vi "Trial v0.vi"(2 "error in (no error)":errorcluster, 3 "queue in":refnum<queue>, 4 "DDA":bool=TRUE) -> (0 "error out":errorcluster={"status"=TRUE, "code"=1, "source"="Enqueue Element in Trial.vi"}, 1 "queue out":refnum<queue>)   [LabVIEW 2017]
uses:
  SubVI/Global.vi
  <vilib>/Analysis/NI_AALPro.lvlib
  <vilib>/robotics/Kinematics/NI_Kinematics.lvlib
  Control/RPY.ctl
  Control/State.ctl
  <vilib>/Analysis/NI_AALBase.lvlib
  <vilib>/Analysis/baseanly.llb/Real Dot Product.vi
  <vilib>/Analysis/_algsub.llb/Real Vector Norm.vi
panel:
  in  "alpha theta":dbl=1.0
  in  "lambda theta":dbl=1.0
  in  "alpha w":dbl=1.0
  in  "lambda w":dbl=1.0
  in  "alpha Rbar":dbl=1.0
  in  "n":i32=2
  in  "Time Target (s)":dbl=10.0
  in  "epsilon":dbl=0.1
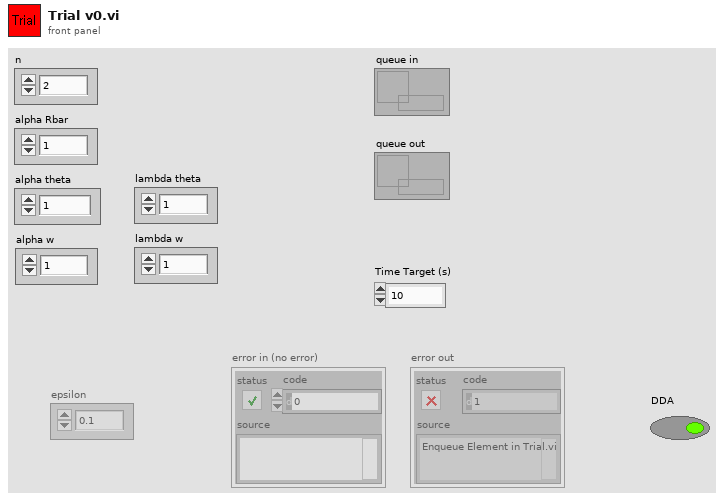
[diagram p1: front panel]
types:
  T1 = typedef "State.ctl" = cluster{"Inertia (Kg)":dbl, "Damping (N*s/m)":dbl, "RoM (deg)":dbl}
  T2 = typedef "RPY.ctl" = cluster{"roll":dbl, "pitch":dbl, "yaw":dbl}
  T3 = typedef "NI_Matrix.lvlib/RealMatrix.ctl" = dbl[][]
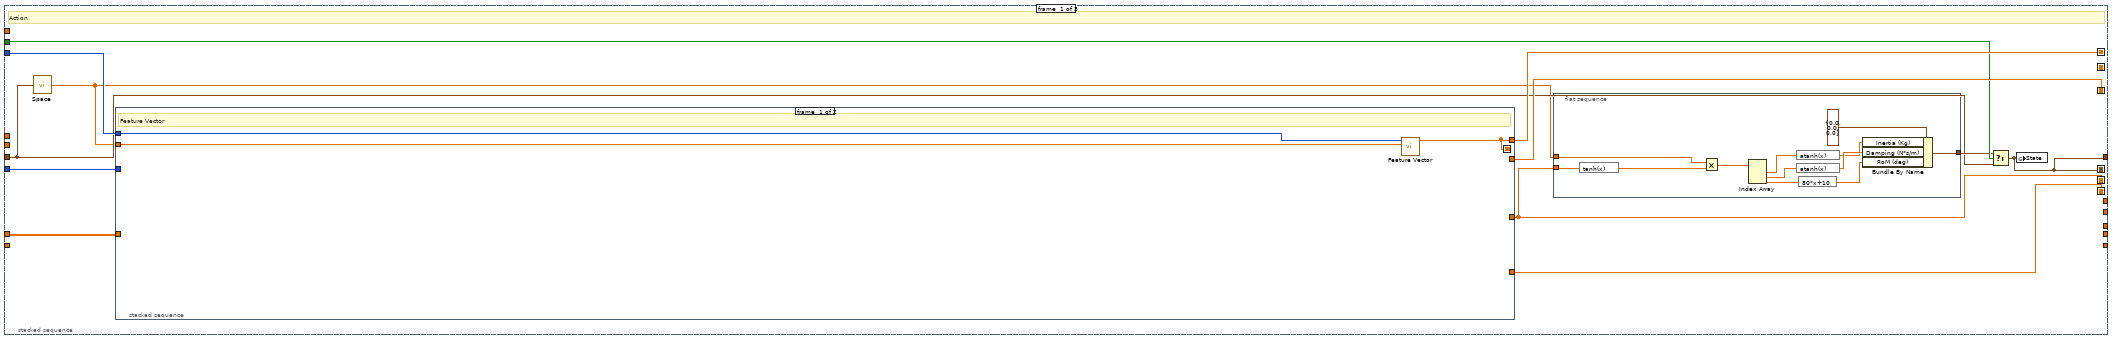
[diagram p7: hidden frame]
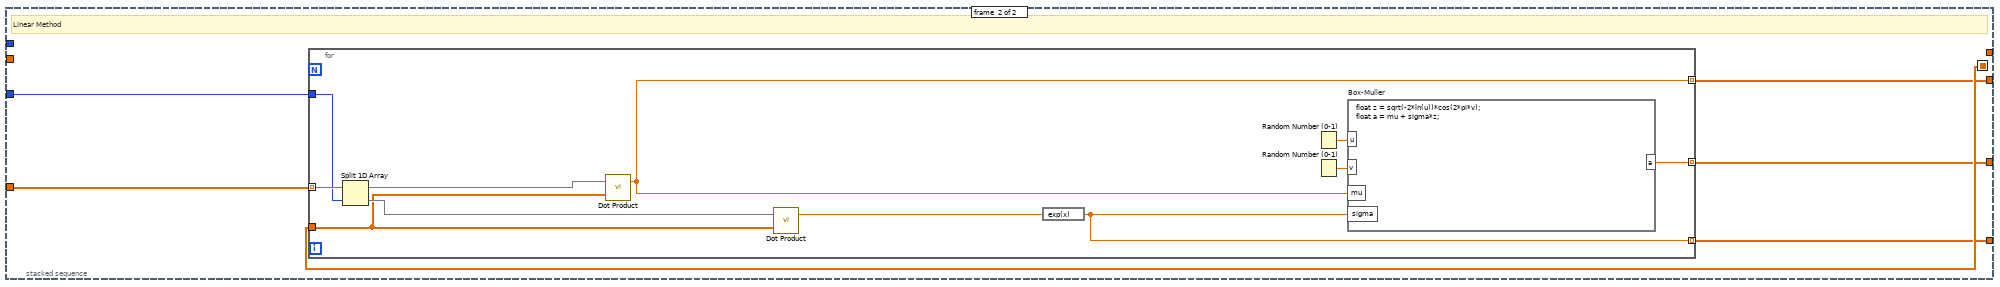
[diagram p8: hidden frame]
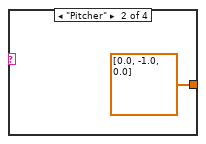
[diagram p9: hidden frame]
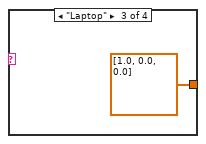
[diagram p10: hidden frame]
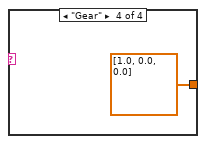
[diagram p11: hidden frame]
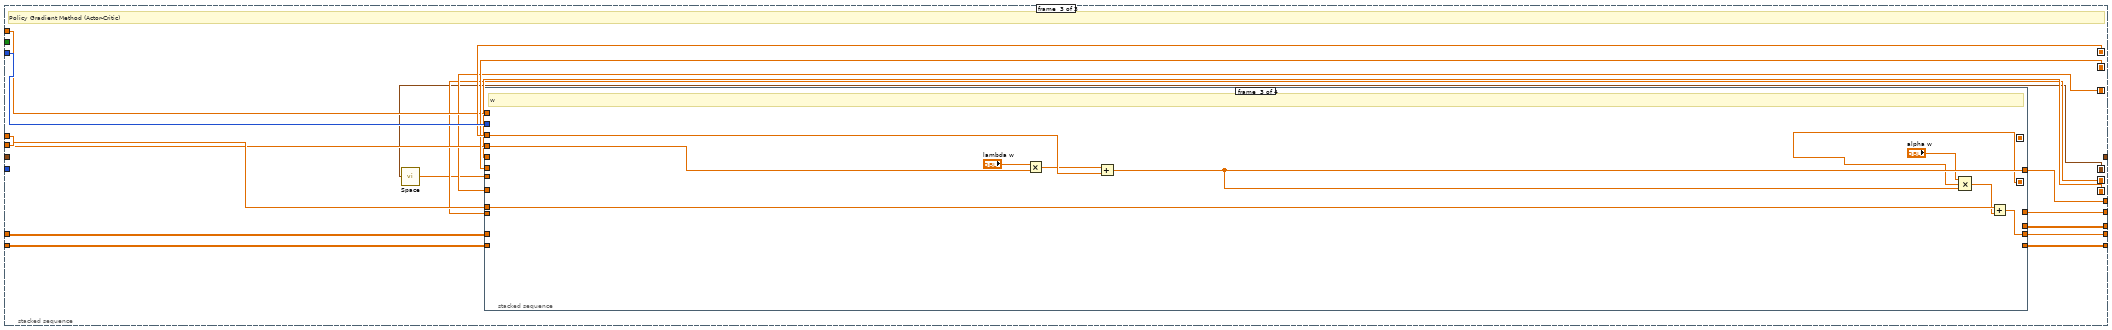
[diagram p12: hidden frame]
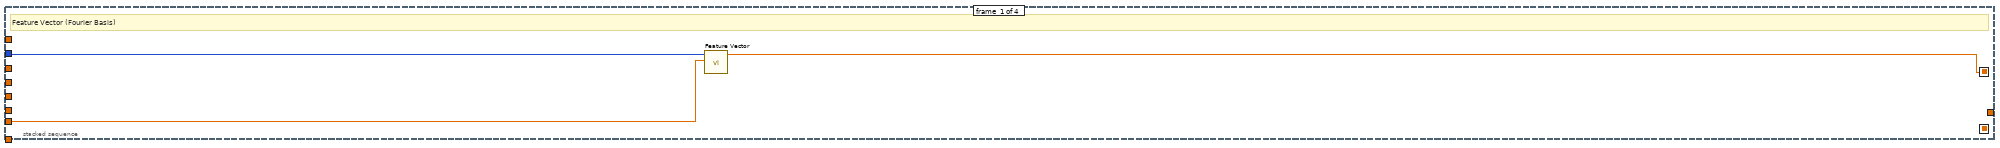
[diagram p13: hidden frame]
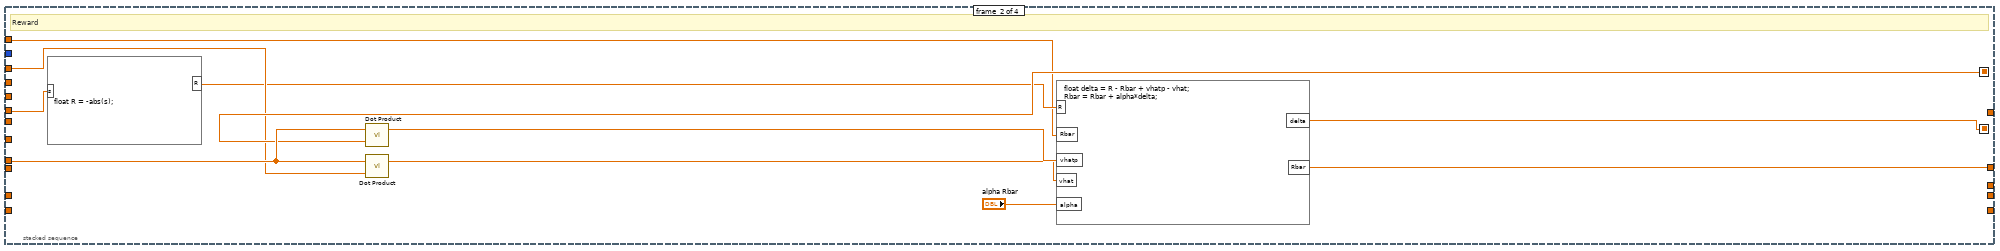
[diagram p14: hidden frame]
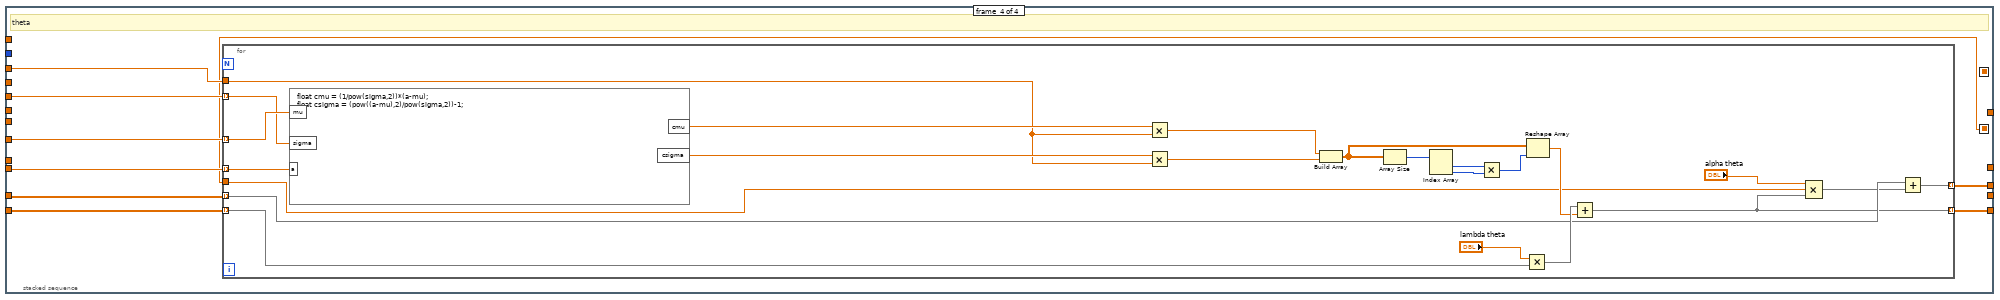
[diagram p15: hidden frame]
diagram:
  n1 = flat-sequence {
    tunnel: [w9] -> w5
    tunnel: "error in (no error)" -> [w10]
    tunnel: "queue in" -> [w8]
    tunnel: "DDA" -> [w11]
    tunnel: [w7] -> w1
    frame #0 {
      w14 = 0.0  # Rbar
      n2 = Increment(x="n") -> (x+1=w18:i32)
      n3 = expression code="2*pow(x,3)"(w18) -> (w20:i32)
      n4 = Initialize Array(0.0 ("element"), 3 ("dimension size"), w20) -> (w12:dbl[][])
      n5 = expression code="pow(x,3)"(w18) -> (w15:i32)
      n6 = Initialize Array(0.0 ("element"), w15) -> (w13:dbl[])
      n7 = global read "Global.vi" "State"() -> (w6:T1)
      n8 = while {
        shift-right: [w37] -> _
        shift-left: w6 -> [w41]
        shift-right: [w28] -> _
        shift-left: w12 -> [w39]
        tunnel: w18 -> [w40]
        tunnel: w15 -> [w38]
        shift-right: [w31] -> _
        shift-left: w13 -> [w36]
        shift-right: [w34] -> _
        shift-left: w14 -> [w35]
        shift-right: [w32] -> _
        shift-left: w13 -> [w33]
        shift-right: [w29] -> _
        shift-left: w12 -> [w30]
        tunnel: w11 -> [w27]
        shift-right: [w23] -> w7
        shift-left: w8 -> [w25]
        shift-right: [w22] -> w9
        shift-left: w10 -> [w26]
        stop <- w42 stop-if-true
        # "Multiple Trials"
        n9 = stacked-sequence {
          seq-local: [w50 _ _] -> [_ w89 w144]
          seq-local: [_ w90 _] -> [_ _ w157]
          seq-local: [w51 _ _] -> [_ _ w159]
          seq-local: [w49 _ _] -> [_ _ w150]
          seq-local: [w48 _ _] -> [_ _ w149]
          seq-local: [w43 _ _] -> [_ _ w148]
          tunnel: w41 -> [w45 _ _]
          tunnel: w40 -> [w54 _ w160]
          tunnel: w39 -> [w53 _ w146]
          tunnel: w38 -> [w52 _ _]
          tunnel: [w50 _ _] -> w37
          tunnel: w36 -> [_ _ w158]
          tunnel: w35 -> [_ _ w156]
          tunnel: [_ _ w155] -> w34
          tunnel: w33 -> [_ _ w154]
          tunnel: [_ _ w153] -> w32
          tunnel: [_ _ w152] -> w31
          tunnel: w30 -> [_ _ w151]
          tunnel: [_ _ w147] -> w29
          tunnel: [_ _ w145] -> w28
          tunnel: w27 -> [w47 _ _]
          frame #0 {
            # "Action"
            n10 = call "Space.vi"("State"=w45) -> ("Array"=w44:dbl[])
            n11 = stacked-sequence {
              seq-local: [w67 _] -> [_ w73]
              tunnel: w54 -> [w69 _]
              tunnel: w53 -> [_ w75]
              tunnel: w52 -> [_ w74]
              tunnel: w44 -> [w68 _]
              tunnel: [w67 _] -> w51
              tunnel: [_ w72] -> w49
              tunnel: [_ w71] -> w48
              tunnel: [_ w70] -> w43
              frame #0 {
                # "Feature Vector"
                n12 = call "Feature Vector.vi"("state"=w68, "n"=w69) -> ("vector"=w67:dbl[])  [unwired: 9 in]
              }
              frame #1 {
                # "Linear Method"
                n13 = for {
                  tunnel: w75 -> [w84] mode=indexing
                  tunnel: w74 -> [w83]
                  tunnel: w73 -> [w80]
                  tunnel: [w78] -> w70 mode=indexing
                  tunnel: [w77] -> w72 mode=indexing
                  tunnel: [w76] -> w71 mode=indexing
                  n14 = Split 1D Array(array=w84, index=w83) -> (first subarray=w82:dbl[], second subarray=w81:dbl[])
                  n15 = call-poly <vilib>:"Dot Product.vi"("Y Vector"=w80, "X Vector"=w82) -> ("X * Y"=w77:dbl)  [unwired: 1 out]
                  n16 = call-poly <vilib>:"Dot Product.vi"("Y Vector"=w80, "X Vector"=w81) -> ("X * Y"=w79:dbl)  [unwired: 1 out]
                  n17 = expression code="exp(x)"(w79) -> (w76:dbl)
                  n18 = Random Number (0-1)() -> (number: 0 to 1=w86:dbl)
                  n19 = Random Number (0-1)() -> (number: 0 to 1=w85:dbl)
                  n20 = formula code="float z = sqrt(-2*ln(u))*cos(2*pi*v);\nfloat a = mu + sigma*z;" "Box-Muller"("u"=w86, "v"=w85, "mu"=w77, "sigma"=w76) -> ("a"=w78:dbl)
                }
              }
            }
            n21 = flat-sequence {
              tunnel: [w66] -> w46
              tunnel: w44 -> [w65]
              tunnel: w43 -> [w56]
              frame #0 {
                n22 = expression code="tanh(x)"(w56) -> (w64:dbl[])
                n23 = Multiply(x=w65, y=w64) -> (x*y=w63:dbl[])
                n24 = Index Array(array=w63) -> (element #1=w58:dbl, element #2=w60:dbl, element #3=w62:dbl)  [unwired: 3 in]
                n25 = expression code="atanh(x)"(w58) -> (w57:dbl)
                n26 = expression code="atanh(x)"(w60) -> (w59:dbl)
                n27 = expression code="80*x+10"(w62) -> (w61:dbl)
                n28 = Bundle By Name(cluster=T1 {"Inertia (Kg)"=0.0, "Damping (N*s/m)"=0.0, "RoM (deg)"=0.0} ("State"), "Inertia (Kg)"=w57, "Damping (N*s/m)"=w59, "RoM (deg)"=w61) -> (w66:T1)
              }
            }
            n29 = Select(t=w46, s=w47, f=w45) -> (s? t:f=w50:T1)
            n30 = global write "Global.vi" "State"(w50) -> ()
          }
          frame #1 {
            # "Observation"
            n31 = global read "Global.vi" "ADL"() -> (w92:string)
            n32 = case shown="\"Book\", Default" w92 {
              tunnel: [dbl[] [0.0, 1.0, 0.0] dbl[] [0.0, -1.0, 0.0] dbl[] [1.0, 0.0, 0.0] dbl[] [1.0, 0.0, 0.0]] -> w91
              frame "Book", Default {
              }
              frame "Pitcher" {
              }
              frame "Laptop" {
              }
              frame "Gear" {
              }
            }
            n33 = Unbundle By Name(w89) -> ("RoM (deg)"=w88:dbl)
            n34 = expression code="(x/180.0)*pi" "degrees to radians"(w88) -> (w87:dbl)
            n35 = call <vilib>:"Angle Vector to Rotation Matrix.vi"("vector"=w91, "angle"=w87) -> ("rotation matrix"=w95:T3)
            n36 = call <vilib>:"Rotation Matrix to Roll Pitch Yaw.vi"("rotation matrix"=w95) -> ("angles"=w96:cluster{"roll":dbl, "pitch":dbl, "yaw":dbl})
            n37 = Unbundle By Name(w96) -> ("roll"=w97:dbl, "pitch"=w98:dbl, "yaw"=w99:dbl)
            n38 = Bundle By Name(cluster=T2 {"roll"=0.0, "pitch"=0.0, "yaw"=0.0} ("Target"), "roll"=w97, "pitch"=w98, "yaw"=w99) -> (w93:T2)
            n39 = while {
              tunnel: w93 -> [w115]
              shift-right: [w107] -> _
              shift-left: 0.0 -> [w108]
              tunnel: [w106] -> _
              tunnel: [w105] -> w90
              i -> [w118]
              stop <- w111 stop-if-true
              # "1 Trial"
              n40 = Quotient & Remainder(x=w118, y=2) -> (x-y*floor(x/y)=w116:i32)  [unwired: 1 out]
              n41 = Equal To 0?(x=w116) -> (x = 0?=w110:bool)
              n42 = Not(x=w110) -> (.not. x?=w109:bool)
              n43 = global read "Global.vi" "Stop"() -> (w112:bool)
              n44 = Select(t=w115, s=w110, f=T2 {"roll"=0.0, "pitch"=0.0, "yaw"=0.0} ("Target")) -> (s? t:f=w113:T2)
              n45 = global write "Global.vi" "Target"(w113) -> ()
              n46 = Or(x=w109, y=w112) -> (x .or. y?=w111:bool)
              n47 = call <vilib>:"High Resolution Relative Seconds.vi"() -> ("relative seconds"=w120:dbl)
              n48 = while {
                tunnel: w113 -> [w127]
                shift-right: [w133] -> _
                shift-left: w120 -> [w134]
                shift-right: [w125] -> _
                shift-left: 0.0 -> [w132]
                tunnel: w108 -> [w126]
                tunnel: [w123] -> w107
                tunnel: ["epsilon"] -> w106
                tunnel: [w122] -> w105
                stop <- w135 stop-if-true
                # "1/2 Trial"
                n49 = Wait (ms)(milliseconds to wait=u32 10) -> ()  [unwired: 1 out]
                n50 = global read "Global.vi" "Object"() -> (w140:T2)
                n51 = call <vilib>:"High Resolution Relative Seconds.vi"() -> ("relative seconds"=w133:dbl)
                n52 = global read "Global.vi" "Playback"() -> (w131:bool)
                n53 = Subtract(x=w140, y=w127) -> (x-y=w141:T2)
                n54 = Subtract(x=w133, y=w134) -> (x-y=w130:dbl)
                n55 = Cluster To Array(cluster=w141) -> (array=w142:dbl[])
                n56 = Select(t=w130, s=w131, f=0.0) -> (s? t:f=w129:dbl)
                n57 = call-poly <vilib>:"Vector Norm.vi"("Input Vector"=w142) -> ("norm"=w139:dbl)  [unwired: 9 in, 1 out]
                n58 = Add(x=w129, y=w132) -> (x+y=w125:dbl)
                n59 = Less?(x=w139, y="epsilon") -> (x < y?=w138:bool)
                n60 = Add(x=w125, y=w126) -> (x+y=w123:dbl)
                n61 = global read "Global.vi" "Stop"() -> (w137:bool)
                n62 = Subtract(x="Time Target (s)", y=w123) -> (x-y=w122:dbl)
                n63 = global write "Global.vi" "Score"(w122) -> ()
                n64 = Or(x=w138, y=w137) -> (x .or. y?=w135:bool)
              }
            }
          }
          frame #2 {
            # "Policy Gradient Method (Actor-Critic)"
            n65 = call "Space.vi"("State"=w144) -> ("Array"=w143:dbl[])
            n66 = stacked-sequence {
              seq-local: [w161 _ _ _] -> [_ w173 _ _]
              seq-local: [_ w164 _ _] -> [_ _ w177 w185]
              tunnel: w143 -> [w163 _ _ _]
              tunnel: w160 -> [w162 _ _ _]
              tunnel: w159 -> [_ w172 w184 w189]
              tunnel: w158 -> [_ w174 w180 _]
              tunnel: w157 -> [_ w169 _ _]
              tunnel: w156 -> [_ w167 _ _]
              tunnel: [_ w165 _ _] -> w155
              tunnel: w154 -> [_ _ w183 _]
              tunnel: [_ _ w178 _] -> w153
              tunnel: [_ _ w175 _] -> w152
              tunnel: w151 -> [_ _ _ w193]
              tunnel: w150 -> [_ _ _ w192]
              tunnel: w149 -> [_ _ _ w191]
              tunnel: w148 -> [_ _ _ w190]
              tunnel: [_ _ _ w188] -> w147
              tunnel: w146 -> [_ _ _ w187]
              tunnel: [_ _ _ w186] -> w145
              frame #0 {
                # "Feature Vector (Fourier Basis)"
                n67 = call "Feature Vector.vi"("state"=w163, "n"=w162) -> ("vector"=w161:dbl[])  [unwired: 9 in]
              }
              frame #1 {
                # "Reward"
                n68 = formula code="float R = -abs(s);"("s"=w169) -> ("R"=w168:dbl)
                n69 = call-poly <vilib>:"Dot Product.vi"("Y Vector"=w173, "X Vector"=w174) -> ("X * Y"=w171:dbl)  [unwired: 1 out]
                n70 = call-poly <vilib>:"Dot Product.vi"("Y Vector"=w172, "X Vector"=w174) -> ("X * Y"=w170:dbl)  [unwired: 1 out]
                n71 = formula code="float delta = R - Rbar + vhatp - vhat;\nRbar = Rbar + alpha*delta;"("R"=w168, "Rbar"=w167, "vhatp"=w171, "vhat"=w170, "alpha"="alpha Rbar") -> ("delta"=w164:dbl, "Rbar"=w165:dbl)
              }
              frame #2 {
                # "w"
                n72 = Multiply(x="lambda w", y=w183) -> (x*y=w181:dbl[])
                n73 = Add(x=w181, y=w184) -> (x+y=w178:dbl[])
                n74 = Compound Arithmetic op=MULTIPLY("alpha w", w177, w178) -> (w179:dbl[])
                n75 = Add(x=w180, y=w179) -> (x+y=w175:dbl[])
              }
              frame #3 {
                # "theta"
                n76 = for {
                  tunnel: w193 -> [w215] mode=indexing
                  tunnel: w192 -> [w213] mode=indexing
                  tunnel: w191 -> [w212] mode=indexing
                  tunnel: w190 -> [w211] mode=indexing
                  tunnel: w189 -> [w208]
                  tunnel: [w198] -> w188 mode=indexing
                  tunnel: w187 -> [w203] mode=indexing
                  tunnel: [w201] -> w186 mode=indexing
                  tunnel: w185 -> [w199]
                  n77 = formula code="float cmu = (1/pow(sigma,2))*(a-mu);\nfloat csigma = (pow((a-mu),2)/pow(sigma,2))-1;"("mu"=w213, "sigma"=w212, "a"=w211) -> ("cmu"=w210:dbl, "csigma"=w209:dbl)
                  n78 = Multiply(x=w210, y=w208) -> (x*y=w207:dbl[])
                  n79 = Multiply(x=w209, y=w208) -> (x*y=w206:dbl[])
                  n80 = Build Array(w207, w206) -> (w197:dbl[][])
                  n81 = Array Size(array=w197) -> (size(s)=w205:i32[])
                  n82 = Index Array(array=w205) -> (element #1=w196:i32, element #2=w195:i32)  [unwired: 2 in]
                  n83 = Multiply(x=w196, y=w195) -> (x*y=w194:i32)
                  n84 = Multiply(x="lambda theta", y=w215) -> (x*y=w214:dbl[])
                  n85 = Reshape Array(w197, w194) -> (w204:dbl[])
                  n86 = Add(x=w214, y=w204) -> (x+y=w198:dbl[])
                  n87 = Compound Arithmetic op=MULTIPLY("alpha theta", w199, w198) -> (w202:dbl[])
                  n88 = Add(x=w203, y=w202) -> (x+y=w201:dbl[])
                }
              }
            }
          }
        }
        n89 = Enqueue Element(queue=w25, element="", error in (no error)=w26) -> (queue out=w23:refnum<queue>, error out=w22:errorcluster)  [unwired: 1 in, 1 out]
        n90 = global read "Global.vi" "Stop"() -> (w42:bool)
      }
    }
  }
  n91 = disable-structure shown="Disabled" {
    frame Disabled {
      n92 = In Range and Coerce(upper limit=90.0, lower limit=0.0) -> (coerced(x)=w226:dbl)  [unwired: 1 in, 1 out]
      n93 = In Range and Coerce(upper limit=inf, lower limit=0.0) -> (coerced(x)=w224:dbl)  [unwired: 1 in, 1 out]
      n94 = In Range and Coerce(upper limit=inf, lower limit=0.0) -> (coerced(x)=w225:dbl)  [unwired: 1 in, 1 out]
      n95 = Bundle By Name(cluster=T1 {"Inertia (Kg)"=0.0, "Damping (N*s/m)"=0.0, "RoM (deg)"=0.0} ("State"), "Inertia (Kg)"=w224, "Damping (N*s/m)"=w225, "RoM (deg)"=w226) -> ()  [unwired: 1 out]
      n96 = Index Array() -> ()  [unwired: 4 in, 3 out]
    }
    frame Enabled {
    }
  }
  n97 = disable-structure shown="Disabled" {
    frame Disabled {
      n98 = expression code="exp(x)"() -> (w229:dbl[])  [unwired: 1 in]
      n99 = Add Array Elements(numeric array=w229) -> (sum=w230:dbl)
      n100 = Divide(x=w229, y=w230) -> (x/y=w227:dbl[])
      n101 = Random Number (0-1)() -> (number: 0 to 1=w231:dbl)
      n102 = for {
        shift-right: [w237] -> _
        shift-left: 0.0 -> [w238]
        tunnel: w231 -> [w236]
        tunnel: [w235] -> w232 mode=indexing
        tunnel: w227 -> [w234] mode=indexing
        n103 = Add(x=w234, y=w238) -> (x+y=w237:dbl)
        n104 = In Range and Coerce(upper limit=w237, x=w236, lower limit=w238) -> (In Range?=w235:bool)  [unwired: 1 out]
      }
      n105 = Boolean To (0,1)(Boolean=w232) -> (0, 1=w233:i16[])
      n106 = To Double Precision Float(number=w233) -> ()  [unwired: 1 out]
    }
    frame Enabled {
    }
  }
  n107 = disable-structure shown="Disabled" {
    frame Disabled {
      n108 = case shown="True" {
        selector: _ -> [_ _]
        frame False {
        }
        frame True {
          # "Policy Gradient Method (Actor-Critic)"
          n109 = stacked-sequence {
            seq-local: [w239 _] -> [_ _]
            frame #0 {
              # "Reward"
              n110 = formula code="float R; //reward\nR = exp(-score);"() -> ("R"=w239:dbl)  [unwired: 1 in]
            }
            frame #1 {
            }
          }
        }
      }
    }
    frame Enabled {
    }
  }
  "error out" <- w5
  "queue out" <- w1
